vi "TestCellUtil.vi"() -> ()   [LabVIEW 2013]
doc: "This setup utility detects the NI Embedded Evaluation Kit hardware on your network and tests the configuration."
uses:
  types/TabStateType.ctl
  Controls/Refs.ctl
  Controls/Button Refs.ctl
  Controls/Tab Ctl Refs.ctl
  Controls/Indicator Refs.ctl
  Controls/Slider Refs.ctl
  Controls/Control Refs.ctl
  Controls/Network Settings.ctl
  types/UserStateType.ctl
  types/ExecutionStateType.ctl
  Controls/Detected.ctl
  Controls/Targets.ctl
  types/MAX Sys Cfg Target Information.ctl
  types/ButtonStateType.ctl
  globals/Globals.vi
  <vilib>/Platform/browser.llb/Open URL in Default Browser (string).vi
  <vilib>/regexp/Match Regular Expression.xnode
panel:
  in  "Tab Control":T1
  out "Welcome":string="Welcome to the Test Cell Controller Setup"
  out "Welcome Message":string="This wizard helps to ensure that your hardware is connected and configured properly to be used as a target in a NI VeriStand system definition.\n\n\nNote: During setup and also during the tutorials, your firewall software may prompt you to block or unblock the National Instruments software.  Select unblock whenever you encounter this prompt."
  out "Instructions":string="Connect Your Test Cell Controller Hardware"
  out "Instructions 2":string="1. Connect the Ethernet cable.\n2. Connect the power cable and press the power button.\n3. Ensure the power LED is on.\n4. Wait 20 seconds for the Test Cell Controller to boot."
  out "Detect Message":string="Click the button below to find the hardware you just connected."
  in  "Begin Detection":bool
  out "Detecting":string="Detecting Hardware\n\nSearching for Test Cell Controllers..."
  out "Detecting 2":i8(slide)=1 scale=0.0..20.0
  in  "IP Troubleshoot 2":bool
  in  "Rescan Targets":bool
  out "Detect Result Tabs":T2(tab)=enum."Found 1"
  out "Found 0 Msg":string="1. Ensure your Test Cell Controller is connected properly.\n2. Restart the Test Cell Controller by pressing the reset button (see image to left for reset button location).\n3. Wait 20 seconds for the Test Cell Controller to boot.\n4.  Click Rescan for Targets.\n\nFor troubleshooting tips, click Troubleshoot."
  out "Found 0 Status":string="Detecting Hardware\n\nNo Test Cell Controllers detected."
  out "None Detected":i8(slide)=100 scale=0.0..100.0
  out "Found 1 Msg":string="1. Check the serial number of your Test Cell Controller (see image to left for serial number location).\n2. Verify the serial number displayed here matches that of your Test Cell Controller.\n\nIf the serial number matches, click Next.\nOtherwise, ensure your hardware is connected properly, then click Rescan for Targets."
  out "Found 1 Status":string="Detecting Hardware\n\nOne Test Cell Controller detected!"
  out "Single Detected":i8(slide)=100 scale=0.0..100.0
  out "MAC Address":string
  in  "MAC Addresses":i32(listbox)=1
  out "Found 1 Msg 2":string="1. Check the serial number of your Test Cell Controller (see image to left for serial number location).\n2. Verify a serial number displayed here matches that of your Test Cell Controller.\n3. If a serial number matches, select it and click Next. \n\nOtherwise, ensure that your hardware is connected properly, then click Rescan for Targets."
  out "Found 2+ Status":string="Detecting Hardware\n\nMultiple Test Cell Controllers detected!"
  out "Multi Detected":i8(slide)=100 scale=0.0..100.0
  out "IP Troubleshoot":string="Failure to detect the Test Cell Controller may be due to one or more of the following:\n\n1. The host computer and Test Cell Controller are on different subnets.\n2. An Ethernet switch or router is off or unplugged.\n3. An Ethernet cable is loose or defective.\n4. The Test Cell Controller was unpowered or booting during the scan.\n\nPlease check for these issues, restart the Test Cell Controller by pressing the restart button (see image to left), and wait 20 seconds for the Test Cell Controller to boot.\n\nFor further troubleshooting tips, click Help.\n\nTo retry detection, click Rescan for Targets."
  out "IP Trouble Title":string="Network Troubleshooting Tips"
  out "Deploy Message":string="Software Install Required\n\nSelect Begin Install to install to the target."
  in  "Begin Deployment":bool
  out "Connecting":string="Testing Configuration\n\nDeploying to Test Cell Controller..."
  out "Deploying":i8(slide)=1 scale=0.0..20.0
  out "Symbol":u16(ring)=2
  in  "Warning":string="Warning: Do not assign the same DNS name to multiple targets on a single network"
  out "Current DNS name:":string
  in  "DNSName":string="Test-Cell-Controller"
  in  "Rename":bool
  in  "System Restore 2":bool
  out "Target MAC Address 2":string="2F14A272" caption="MAC Address"
  out "Connecting Done":string="Testing Configuration\n\nTarget software is configured correctly"
  out "Deploy Finish":i8(slide)=100 scale=0.0..100.0
  in  "Launch proj wiz":bool
  out "Complete":string="Setup Complete"
  out "Success 2":string="1. Please record the Test Cell Controller's IP Address (displayed above). It is needed for use in NI VeriStand.\n2. Click Exit Setup and Launch New Project Wizard to create a new Test Cell Controller Project."
  out "IP Address":string="10.0.42.188"
  in  "Help":bool
  out "DHCP Tabs":enum32{"IP Assignment", "DHCP", "Manual IP"}(tab)
  out "Net Setup":string="Networking Setup and Software Installation\n"
  in  "Static IP":bool
  out "DHCP Failed Tab":enum32{"Failed", "Blank"}(tab)=enum."Blank"
  out "IP Err1":string="Go back to Step 2 and check configuration."
  in  "DHCP":bool
  out "Auto IP":string="Automatic: If your Test Cell Controller is connected to your host PC through an Ethernet switch or router, select Automatic IP to request an IP address via DHCP. Contact your network administrator if your network does not support DHCP."
  in  "Default Gateway":string="10.1.128.1"
  in  "DNS Server":string="130.164.12.8"
  in  "Subnet Mask":string="255.255.254.0"
  in  "Target IP Address":string="10.1.128.143"
  out "Manual IP":string="Static (Advanced): If your Test Cell Controller is connected to your host PC directly, enter the appropriate network information below and select Static IP."
  out "Manual IP Failed Tab":enum32{"Failed", "Blank"}(tab)=enum."Blank"
  out "IP Err2":string="Go back to Step 2 and check configuration."
  out "DHCP Message":string="Configuring Test Cell Controller IP Address\n\nAttempting Automatic IP Assignment..."
  out "Assigning Auto":i8(slide)=6 scale=0.0..20.0
  out "Restore Time Note 2":string="Please be patient, this may take several minutes."
  out "Manual IP Message":string="Configuring Test Cell Controller IP Address\n\nAttempting Manual IP Assignment..."
  out "Assigning Manual":i8(slide)=6 scale=0.0..20.0
  out "Restore Time Note 3":string="Please be patient, this may take several minutes."
  out "Trouble Message 2":string="Deployment Failed"
  out "Trouble Warning":string="Restoring the target will erase all existing software on the target and may take several minutes. Please confirm that the serial number below matches the serial number printed on the target to be restored.\n\nNote: To be detected after restoration, the target must be located on the same subnet as the host computer."
  out "Trouble Message":string="1. Please reset the Test Cell Controller (see image below) and wait 20 seconds.\n2. Select Previous, then select Rescan for Targets. \n3. If deployment fails multiple times, select Restore Target System to reformat the Test Cell Controller and reimage it with the necessary software. "
  in  "System Restore":bool
  out "Target MAC Address":string="2F14A272"
  out "Reimage Tabs":enum32{"Running", "Success", "Failure"}(tab)
  out "Restore Time Note":string="Please be patient, this may take several minutes."
  out "Reimaging Tabs":enum32{"Reformat", "Reimage", "IP Config"}(tab)=enum."Reimage"
  out "Reformatting":string="Restoring Test Cell Controller\n\nReformatting ..."
  out "Reimaging":string="Installing Test Cell Controller Software\n\nCopying files ..."
  out "Auto IP Message":string="Configuring Test Cell Controller IP Address\n\nAttempting Automatic IP Assignment..."
  out "Restoring 2":i8(slide)=1 scale=0.0..20.0
  out "Restoring":i8(slide)=3 scale=0.0..20.0
  in  "Redeploy":bool
  out "Reimage Success Msg":string="The Test Cell Controller has been successfully restored."
  out "Reimage Success":string="Installing Test Cell Controller Software\n\nSuccess!"
  out "Install Success":i8(slide)=20 scale=0.0..20.0
  out "Reimage Failure":string="Installing Test Cell Controller Software\n\nFailed."
  out "Restore Failed":i8(slide)=20 scale=0.0..20.0
  out "Reimage Failure Msg":string="Your target did not reimage properly.\nPlease double-check your configuration and then contact support."
  out "Error Details:":errorcluster={"status"=TRUE, "code"=-2147220616, "source"="nisyscfg.lvlib:Get System Experts.vi:1<APPEND>\n\n<b>Complete call chain:</b>\r\n     nisyscfg.lvlib:Get System Experts.vi:1\r\n     nisyscfg.lvlib:Initialize (String).vi:1\r\n     RunDetection.vi\r\n     EvalUtil.vi"}
  out "Generic Error":string="      Unhandled Error Detected\n\nEnsure the Test Cell Controller is connected properly and reset it.  Then select Previous to retry the operation.  If the operation continues to fail, contact National Instruments for support at (866) 275-6964."
  in  "Skip Man":bool
  out "Congrats":string="Congratulations!"
  out "Success 1":string="Your Test Cell Controller has been successfully configured!\n\nIf you are new to using NI VeriStand, select Launch Getting Started Manual.  Otherwise, select Skip Manual."
  in  "GetStart Man":bool
  out "RenamingText":string="Renaming Test Cell Controller\n\nPlease be patient, this may take a minute."
  out "Renaming":i8(slide)=1 scale=0.0..20.0
  out "Main Title":string="National Instruments Test Cell Controller Setup"
  out "Step 5":string="Step 5:\nComplete"
  out "Step 4":string="Step 4:\nTarget Setup"
  out "Step 3":string="Step 3:\nHardware Detection"
  out "Step 2":string="Step 2:\nHardware Setup"
  out "Step 1":string="Step 1:\nWelcome"
  out "Skip deploy":bool
  out "LED 5":bool
  out "LED 4":bool
  out "LED 3":bool
  out "LED 2":bool
  out "LED 1":bool=TRUE
  out "Main Progress":u8(slide) scale=0.0..100.0
  in  "Exit":bool
  in  "Next":bool
  in  "Prev":bool
  in  "error in (no error)":errorcluster
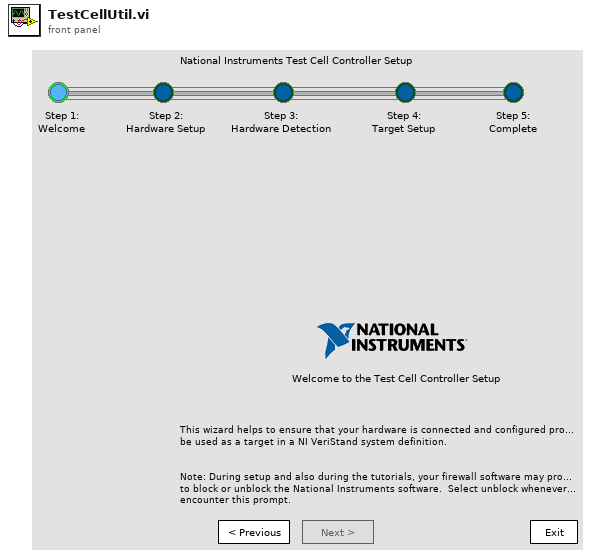
[diagram p1: front panel]
types:
  T1 = typedef "TabStateType.ctl" = enum32{"Welcome", "Instructions", "Detect", "Run Detection", "Detect Result", "Deploy", "Run Deployment", "Connect Verify", "Success", "DHCP", "Troubleshoot", "System Restore", "Error", "Video", "Rename"}
  T2 = enum32{"Found 0", "Found 1", "Found 2", "Found 3"}
  T3 = typedef "Targets.ctl" = cluster{"Dectected":T4, "Filtered Targets":T5[]}
  T4 = typedef "Detected.ctl" = enum16{"None", "Failed", "Single", "Multi"}
  T5 = typedef "MAX Sys Cfg Target Information.ctl" = cluster{"MAC Address":string, "IP Address":string, "Status":string, "Product Name":string, "Hostname":string, "Firmware/Safe Mode":string, "Subnet Mask":string, "Gateway":string, "DNS Server":string, "Serial Number":string, "Product ID":u32, "Locked ":bool, "LocalSubnet":bool, "Halt If TCP/IP Fails":bool, "Password Protected Reset":bool, "IP Mode":i32}
  T6 = typedef "ExecutionStateType.ctl" = enum16{"Init", "Welcome", "Idle", "Detect", "Run Detection", "Detect Fail", "Detect One", "Detect Mult", "Deploy", "DHCP", "Static IP", "Run Deployment", "Connect Verify", "Exit", "Video Wait", "Success", "Troubleshoot", "Troubleshoot 2", "RenameDNS"}
  T7 = typedef "UserStateType.ctl" = enum16{"Welcome", "Instructions", "Detect", "Deploy", "Success"}
  T8 = typedef "Network Settings.ctl" = cluster{"Image by default?":bool, "Working IP Config known?":bool, "DHCP?":bool}
  T9 = typedef "Refs.ctl" = cluster{"Button Refs":T10, "Tab Ctl Refs":T11, "Indicator Refs":T12, "Slider Refs":T13, "Control Refs":T14, "Deploy Message":refnum<vi>}
  T10 = typedef "Button Refs.ctl" = cluster{"Next":refnum<vi>, "Prev":refnum<vi>, "Help":refnum<vi>, "Exit":refnum<vi>, "IP Troubleshoot":refnum<vi>, "Video":refnum<vi>, "Skip Video":refnum<vi>, "Rename":refnum<vi>}
  T11 = typedef "Tab Ctl Refs.ctl" = cluster{"Tab":refnum<vi>, "Detect Result":refnum<vi>, "DHCP":refnum<vi>, "Reimage":refnum<vi>, "Reimaging":refnum<vi>, "Manual IP Failed":refnum<vi>, "DHCP Failed":refnum<vi>}
  T12 = typedef "Indicator Refs.ctl" = cluster{"Main Progress":refnum<vi>, "LED 1":refnum<vi>, "LED 2":refnum<vi>, "LED 3":refnum<vi>, "LED 4":refnum<vi>, "LED 5":refnum<vi>, "MAC Address":refnum<vi>, "Error":refnum<vi>, "Target MAC Address":refnum<vi>, "Target MAC Address 2":refnum<vi>, "IP Address":refnum<vi>, "CurrentDNSName":refnum<vi>, "Symbol":refnum<vi>, "Warning":refnum<vi>}
  T13 = typedef "Slider Refs.ctl" = cluster{"Detecting":refnum<vi>, "Single Detected":refnum<vi>, "Multi Detected":refnum<vi>, "None Detected":refnum<vi>, "Deploying":refnum<vi>, "Deploy Finish":refnum<vi>, "Assigning Manual":refnum<vi>, "Assigning Auto":refnum<vi>, "Restoring":refnum<vi>, "Restoring 2":refnum<vi>, "Restore Success":refnum<vi>, "Restore Failed":refnum<vi>, "Renaming":refnum<vi>}
  T14 = typedef "Control Refs.ctl" = cluster{"MAC Addresses":refnum<vi>, "Target IP Address":refnum<vi>, "Subnet Mask":refnum<vi>, "DNS IP":refnum<vi>, "Default Gateway":refnum<vi>, "DNSName":refnum<vi>}
  T15 = typedef "ButtonStateType.ctl" = enum16{"No change", "No Next", "No Prev", "All Disabled", "All Enabled", "Exit Only"}
  T16 = enum8{"Enabled", "Disabled", "Disabled and Grayed Out"}
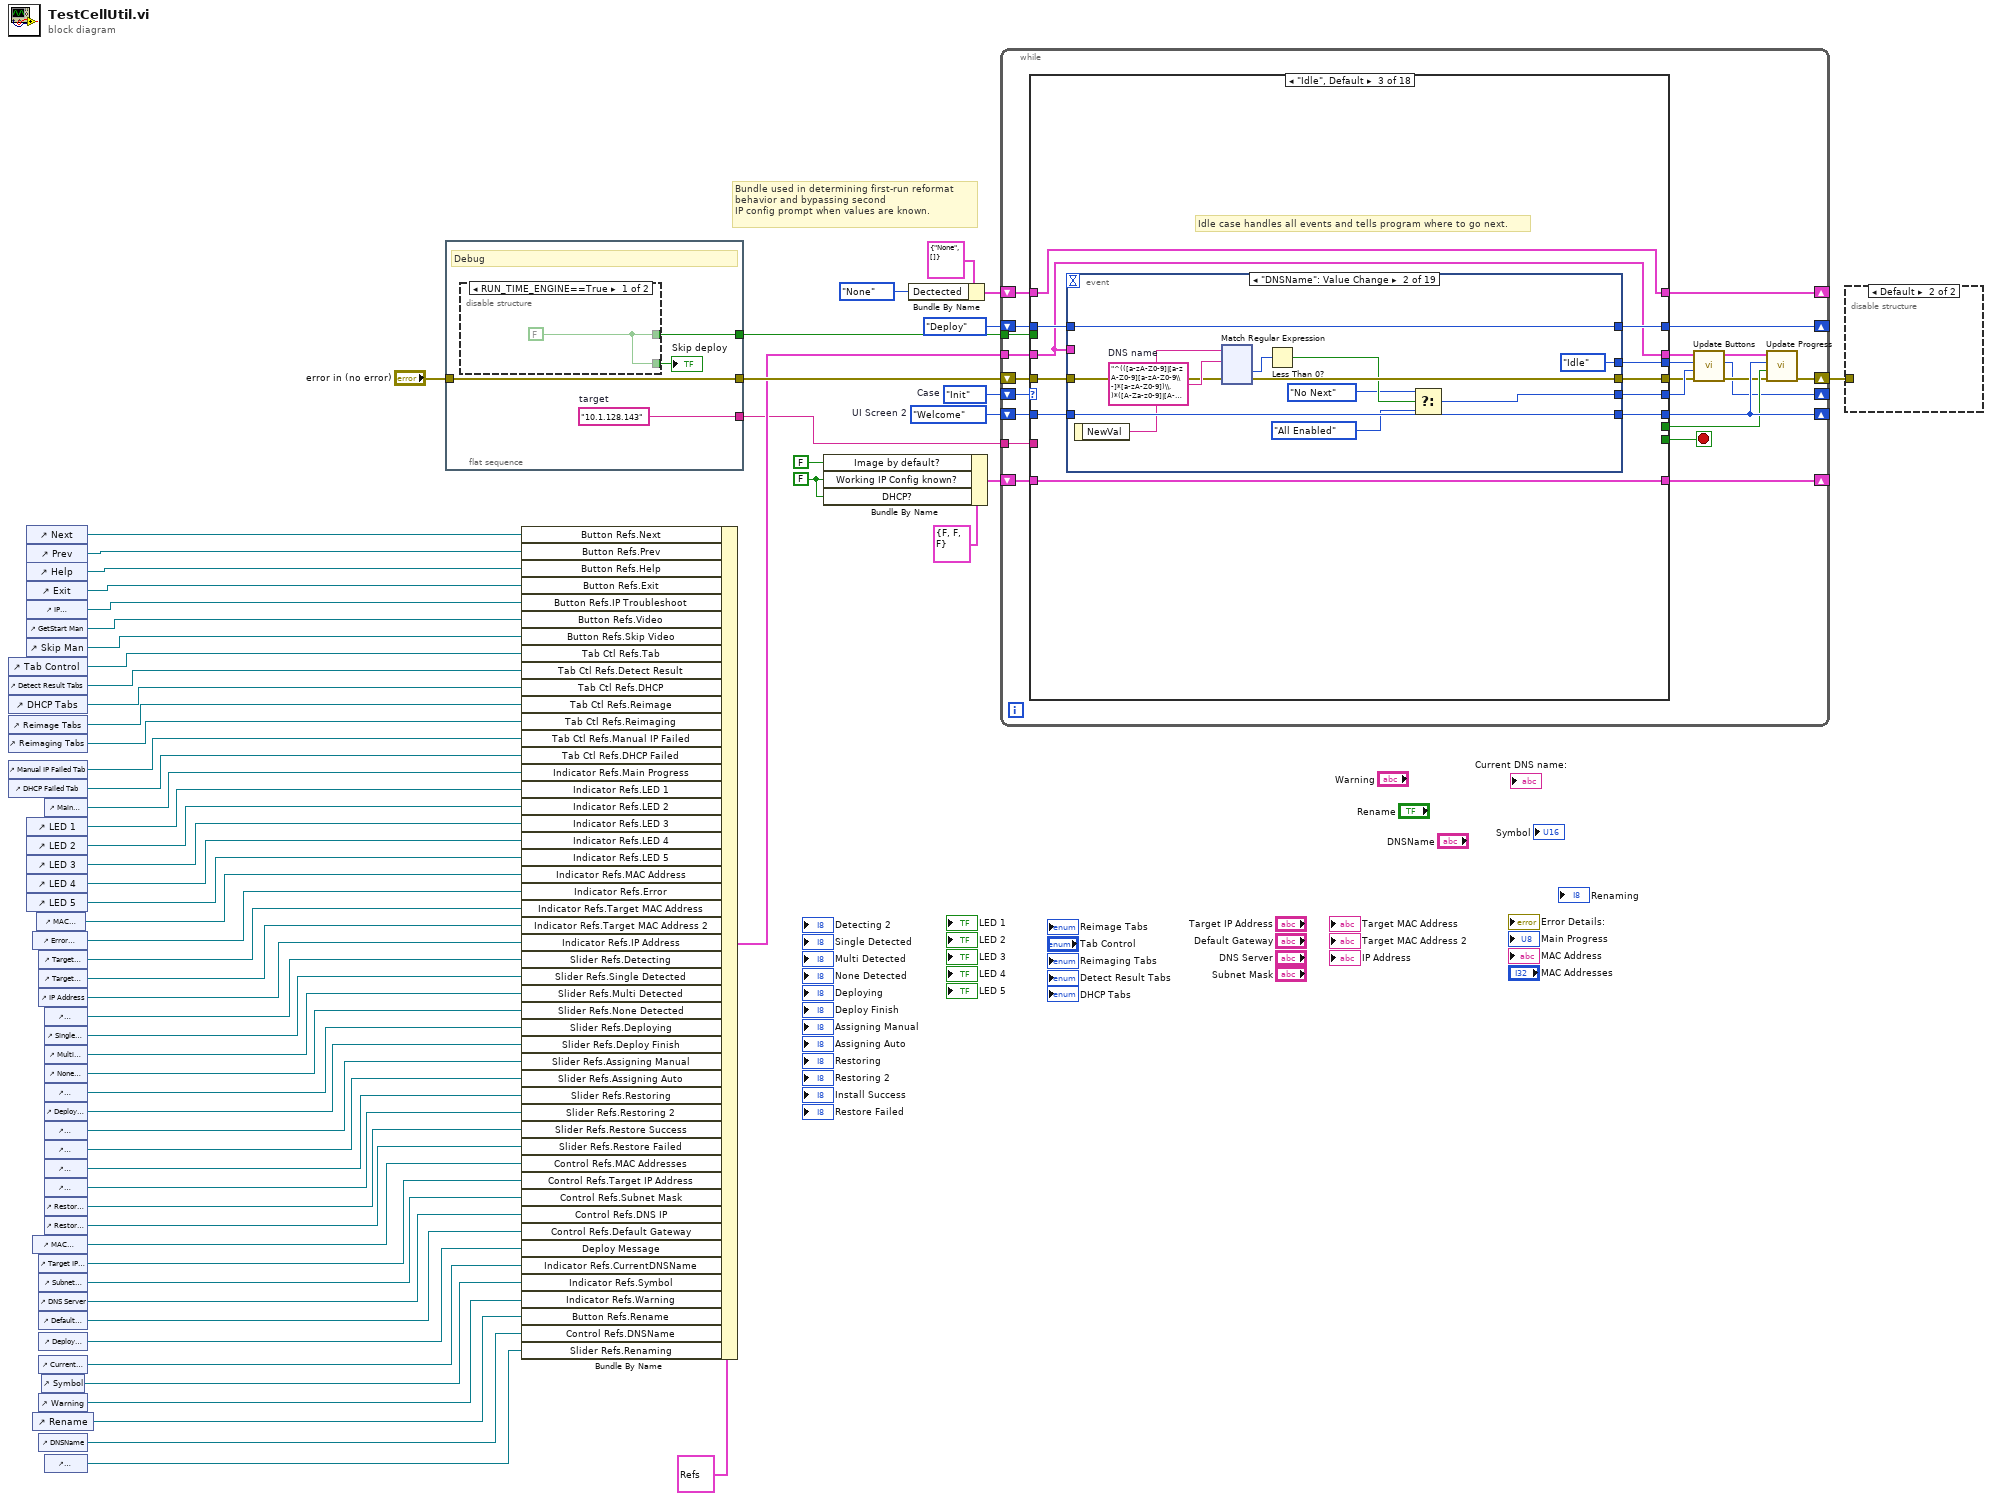
[diagram p0: block diagram]
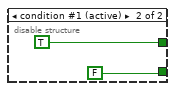
[diagram p2: hidden frame]
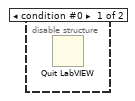
[diagram p3: hidden frame]
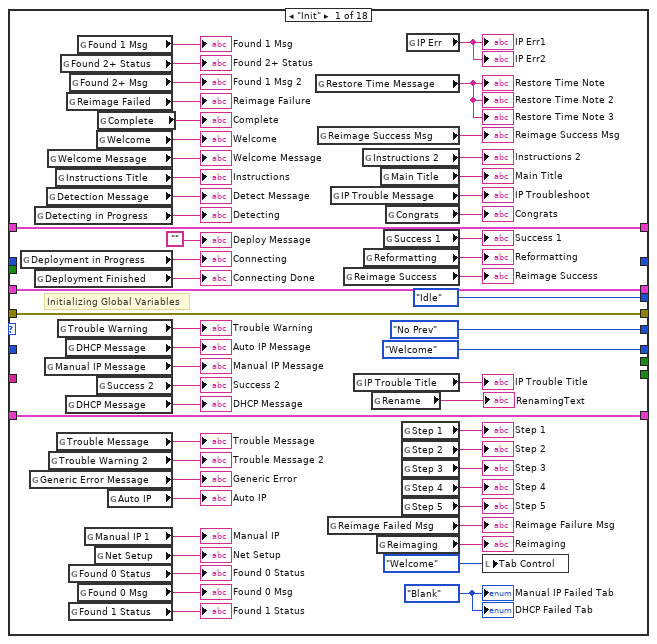
[diagram p4: hidden frame]
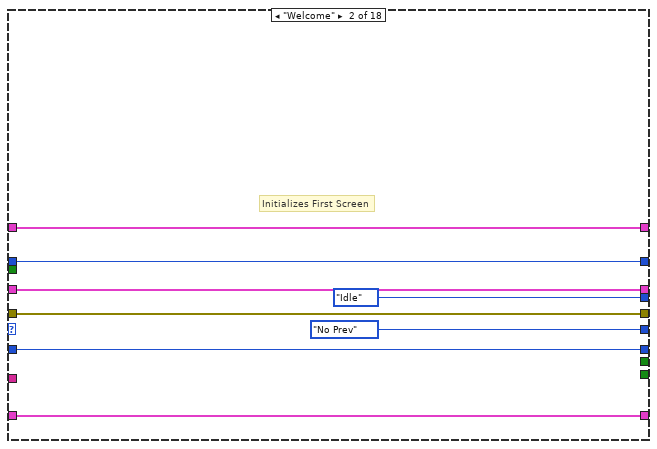
[diagram p5: hidden frame]
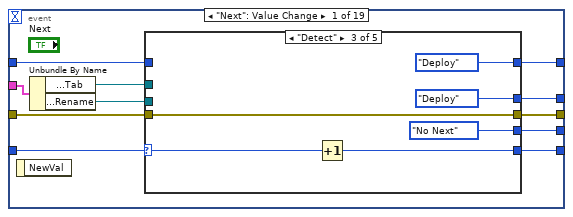
[diagram p6: hidden frame]
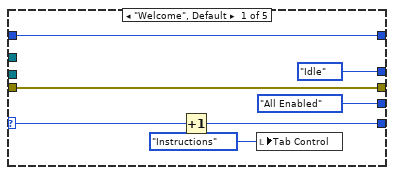
[diagram p7: hidden frame]
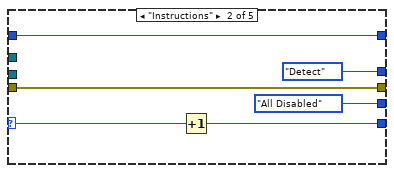
[diagram p8: hidden frame]
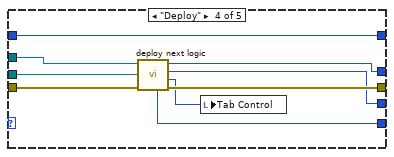
[diagram p9: hidden frame]
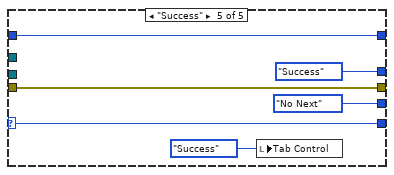
[diagram p10: hidden frame]
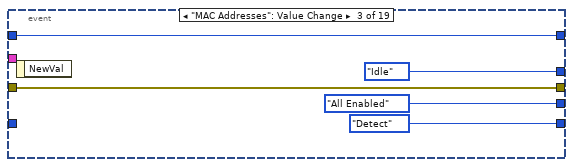
[diagram p11: hidden frame]
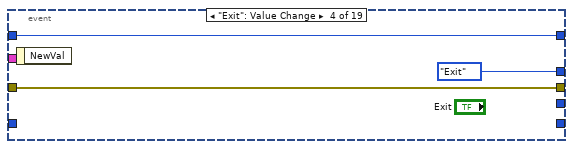
[diagram p12: hidden frame]
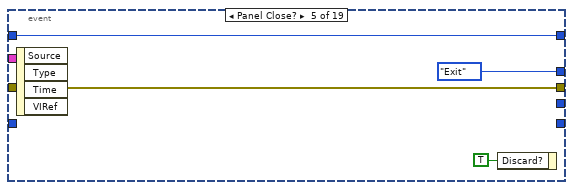
[diagram p13: hidden frame]
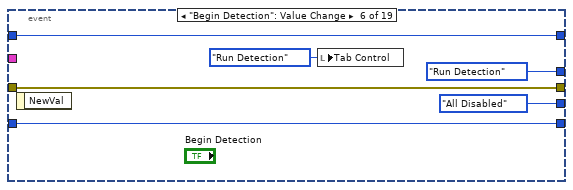
[diagram p14: hidden frame]
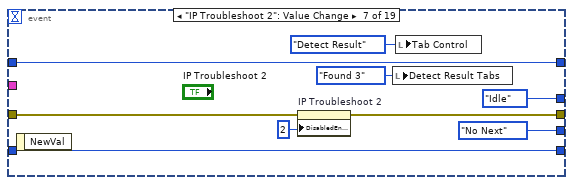
[diagram p15: hidden frame]
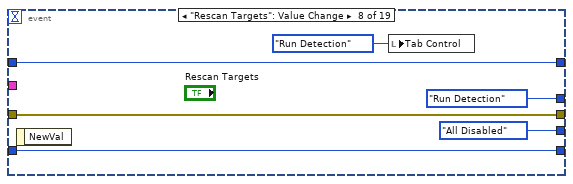
[diagram p16: hidden frame]
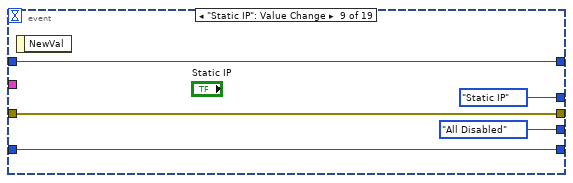
[diagram p17: hidden frame]
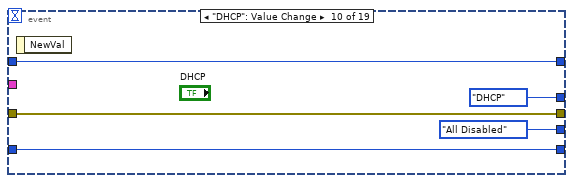
[diagram p18: hidden frame]
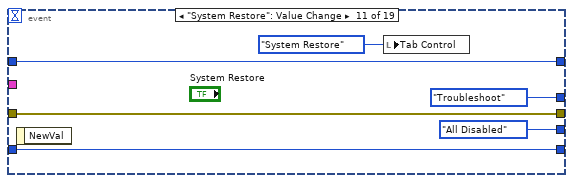
[diagram p19: hidden frame]
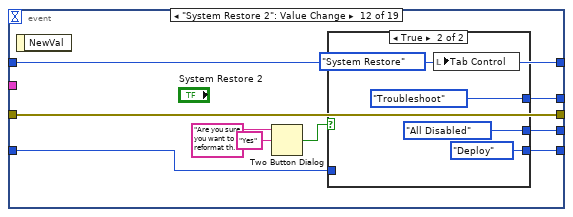
[diagram p20: hidden frame]
diagram:
  w40 = FALSE ("Working IP Config known?")
  w47 = ExecutionStateType."Init"  # Case
  w48 = UserStateType."Welcome"  # UI Screen 2
  # "Image by default?"
  # "Bundle used in determining first-run reformat\nbehavior and bypassing second\nIP config prompt when values are known."
  n1 = control-ref of="Tab Control"() -> (w58:refnum<vi>)
  n2 = control-ref of="Detect Result Tabs"() -> (w57:refnum<vi>)
  n3 = control-ref of="DHCP Tabs"() -> (w56:refnum<vi>)
  n4 = control-ref of="Reimage Tabs"() -> (w7:refnum<vi>)
  n5 = control-ref of="Reimaging Tabs"() -> (w33:refnum<vi>)
  n6 = control-ref of="Manual IP Failed Tab"() -> (w32:refnum<vi>)
  n7 = control-ref of="DHCP Failed Tab"() -> (w31:refnum<vi>)
  n8 = control-ref of="Next"() -> (w65:refnum<vi>)
  n9 = control-ref of="Prev"() -> (w64:refnum<vi>)
  n10 = control-ref of="Help"() -> (w63:refnum<vi>)
  n11 = control-ref of="Exit"() -> (w62:refnum<vi>)
  n12 = control-ref of="IP Troubleshoot 2"() -> (w61:refnum<vi>)
  n13 = control-ref of="GetStart Man"() -> (w60:refnum<vi>)
  n14 = control-ref of="Skip Man"() -> (w59:refnum<vi>)
  n15 = control-ref of="LED 1"() -> (w54:refnum<vi>)
  n16 = control-ref of="LED 2"() -> (w53:refnum<vi>)
  n17 = control-ref of="LED 3"() -> (w52:refnum<vi>)
  n18 = control-ref of="LED 4"() -> (w51:refnum<vi>)
  n19 = control-ref of="LED 5"() -> (w50:refnum<vi>)
  n20 = control-ref of="Error Details:"() -> (w38:refnum<vi>)
  n21 = control-ref of="MAC Addresses"() -> (w17:refnum<vi>)
  n22 = control-ref of="Rename"() -> (w3:refnum<vi>)
  n23 = control-ref of="MAC Address"() -> (w49:refnum<vi>)
  n24 = control-ref of="Target MAC Address"() -> (w20:refnum<vi>)
  n25 = control-ref of="Target MAC Address 2"() -> (w19:refnum<vi>)
  n26 = control-ref of="IP Address"() -> (w18:refnum<vi>)
  n27 = control-ref of="Target IP Address"() -> (w16:refnum<vi>)
  n28 = control-ref of="Subnet Mask"() -> (w15:refnum<vi>)
  n29 = control-ref of="DNS Server"() -> (w14:refnum<vi>)
  n30 = control-ref of="Default Gateway"() -> (w13:refnum<vi>)
  n31 = control-ref of="Deploy Message"() -> (w8:refnum<vi>)
  n32 = control-ref of="Current DNS name:"() -> (w6:refnum<vi>)
  n33 = control-ref of="Warning"() -> (w4:refnum<vi>)
  n34 = control-ref of="DNSName"() -> (w2:refnum<vi>)
  n35 = control-ref of="Symbol"() -> (w5:refnum<vi>)
  n36 = control-ref of="Main Progress"() -> (w55:refnum<vi>)
  n37 = control-ref of="Detecting 2"() -> (w12:refnum<vi>)
  n38 = control-ref of="Single Detected"() -> (w30:refnum<vi>)
  n39 = control-ref of="Multi Detected"() -> (w29:refnum<vi>)
  n40 = control-ref of="None Detected"() -> (w28:refnum<vi>)
  n41 = control-ref of="Deploying"() -> (w27:refnum<vi>)
  n42 = control-ref of="Deploy Finish"() -> (w26:refnum<vi>)
  n43 = control-ref of="Assigning Manual"() -> (w25:refnum<vi>)
  n44 = control-ref of="Assigning Auto"() -> (w24:refnum<vi>)
  n45 = control-ref of="Restoring"() -> (w23:refnum<vi>)
  n46 = control-ref of="Restoring 2"() -> (w9:refnum<vi>)
  n47 = control-ref of="Restore Success"() -> (w22:refnum<vi>)
  n48 = control-ref of="Restore Failed"() -> (w21:refnum<vi>)
  n49 = control-ref of="Renaming"() -> (w1:refnum<vi>)
  n50 = flat-sequence {
    tunnel: [w70] -> w44
    tunnel: "error in (no error)" -> [w70]
    tunnel: [w68] -> w11
    tunnel: [w69] -> w10
    frame #0 {
      w69 = "10.1.128.143"  # target
      # "Debug"
      n51 = disable-structure shown="RUN_TIME_ENGINE==True" {
        disable-tunnel: [w71 TRUE ("Software-Only?")] -> w68
        disable-tunnel: [w71 FALSE ("Skip deploy")] -> w67
        frame condition #0 {
          w71 = FALSE ("Software-Only?")
        }
        frame condition #1 (active) {
        }
      }
      "Skip deploy" <- w67
    }
  }
  n52 = Bundle By Name(cluster=T9 {"Button Refs"={"Next"=refnum, "Prev"=refnum, "Help"=refnum, "Exit"=refnum, "IP Troubleshoot"=refnum, "Video"=refnum, "Skip Video"=refnum, "Rename"=refnum}, "Tab Ctl Refs"={"Tab"=refnum, "Detect Result"=refnum, "DHCP"=refnum, "Reimage"=refnum, "Reimaging"=refnum, "Manual IP Failed"=refnum, "DHCP Failed"=refnum}, "Indicator Refs"={"Main Progress"=refnum, "LED 1"=refnum, "LED 2"=refnum, "LED 3"=refnum, "LED 4"=refnum, "LED 5"=refnum, "MAC Address"=refnum, "Error"=refnum, "Target MAC Address"=refnum, "Target MAC Address 2"=refnum, "IP Address"=refnum, "CurrentDNSName"=refnum, "Symbol"=refnum, "Warning"=refnum}, "Slider Refs"={"Detecting"=refnum, "Single Detected"=refnum, "Multi Detected"=refnum, "None Detected"=refnum, "Deploying"=refnum, "Deploy Finish"=refnum, "Assigning Manual"=refnum, "Assigning Auto"=refnum, "Restoring"=refnum, "Restoring 2"=refnum, "Restore Success"=refnum, "Restore Failed"=refnum, "Renaming"=refnum}, "Control Refs"={"MAC Addresses"=refnum, "Target IP Address"=refnum, "Subnet Mask"=refnum, "DNS IP"=refnum, "Default Gateway"=refnum, "DNSName"=refnum}, "Deploy Message"=refnum} ("Ctl Refs"), "Button Refs.Next"=w65, "Button Refs.Prev"=w64, "Button Refs.Help"=w63, "Button Refs.Exit"=w62, "Button Refs.IP Troubleshoot"=w61, "Button Refs.Video"=w60, "Button Refs.Skip Video"=w59, "Tab Ctl Refs.Tab"=w58, "Tab Ctl Refs.Detect Result"=w57, "Tab Ctl Refs.DHCP"=w56, "Tab Ctl Refs.Reimage"=w7, "Tab Ctl Refs.Reimaging"=w33, "Tab Ctl Refs.Manual IP Failed"=w32, "Tab Ctl Refs.DHCP Failed"=w31, "Indicator Refs.Main Progress"=w55, "Indicator Refs.LED 1"=w54, "Indicator Refs.LED 2"=w53, "Indicator Refs.LED 3"=w52, "Indicator Refs.LED 4"=w51, "Indicator Refs.LED 5"=w50, "Indicator Refs.MAC Address"=w49, "Indicator Refs.Error"=w38, "Indicator Refs.Target MAC Address"=w20, "Indicator Refs.Target MAC Address 2"=w19, "Indicator Refs.IP Address"=w18, "Slider Refs.Detecting"=w12, "Slider Refs.Single Detected"=w30, "Slider Refs.Multi Detected"=w29, "Slider Refs.None Detected"=w28, "Slider Refs.Deploying"=w27, "Slider Refs.Deploy Finish"=w26, "Slider Refs.Assigning Manual"=w25, "Slider Refs.Assigning Auto"=w24, "Slider Refs.Restoring"=w23, "Slider Refs.Restoring 2"=w9, "Slider Refs.Restore Success"=w22, "Slider Refs.Restore Failed"=w21, "Control Refs.MAC Addresses"=w17, "Control Refs.Target IP Address"=w16, "Control Refs.Subnet Mask"=w15, "Control Refs.DNS IP"=w14, "Control Refs.Default Gateway"=w13, "Deploy Message"=w8, "Indicator Refs.CurrentDNSName"=w6, "Indicator Refs.Symbol"=w5, "Indicator Refs.Warning"=w4, "Button Refs.Rename"=w3, "Control Refs.DNSName"=w2, "Slider Refs.Renaming"=w1) -> (w34:T9)
  n53 = Bundle By Name(cluster=T8 {"Image by default?"=FALSE, "Working IP Config known?"=FALSE, "DHCP?"=FALSE} ("Network Settings"), "Image by default?"=FALSE, "Working IP Config known?"=w40, "DHCP?"=w40) -> (w39:T8)
  n54 = Bundle By Name(cluster=T3 {"Dectected"=enum."None", "Filtered Targets"=[]} ("Targets"), "Dectected"=Detected."None") -> (w35:T3)
  n55 = while {
    shift-right: [w82] -> w43
    shift-left: w44 -> [w96]
    shift-right: [w89] -> _
    shift-left: w48 -> [w95]
    shift-right: [w77] -> _
    shift-left: w47 -> [w74]
    shift-right: [w81] -> _
    shift-left: w35 -> [w94]
    shift-right: [w92] -> _
    shift-left: enum16{"Deploy", "Troubleshoot"}."Deploy" -> [w93]
    shift-right: [w78] -> _
    shift-left: w39 -> [w90]
    tunnel: w34 -> [w80]
    tunnel: w11 -> [w76]
    tunnel: w10 -> [w75]
    stop <- w91 stop-if-true
    n56 = case shown="\"Idle\", Default" w74 {
      selector: w74 -> [_ _ _ _ _ _ _ _ _ w569 _ _ _ _ _ _ _ _]
      tunnel: [UserStateType."Welcome" ("Enum 2") w156 w170 UserStateType."Detect" ("Enum 2") w516 w529 w538 w549 UserStateType."Deploy" ("Enum 2") UserStateType."Deploy" ("Enum 2") UserStateType."Deploy" ("Enum 2") w593 w600 w609 w620 UserStateType."Deploy" ("Enum 2") w641 w646] -> w89
      tunnel: w96 -> [w99 w159 w169 w502 w517 w527 w537 w548 w559 w574 w584 w588 w595 w604 w617 w634 w644 w655]
      tunnel: [w99 w159 w168 w504 w515 w526 w534 w543 w562 w572 w585 w587 w595 w605 w616 w631 w643 w654] -> w83
      tunnel: [_ _ _ _ _ _ _ _ _ _ _ _ TRUE _ _ _ _ _] -> w91
      tunnel: [ButtonStateType."No Prev" ("Enum") ButtonStateType."No Prev" ("Enum") w167 ButtonStateType."All Disabled" ("Enum") ButtonStateType."All Disabled" ("Enum") w525 ButtonStateType."All Enabled" ("Enum") ButtonStateType."No Next" ("Enum") w560 w573 w582 w591 ButtonStateType."No Next" ("Enum") ButtonStateType."No Next" ("Enum") ButtonStateType."No change" ("Enum") w630 ButtonStateType."No Next" ("Enum") w648] -> w85
      tunnel: w95 -> [_ w156 w166 _ w516 w529 w538 w549 _ _ _ w593 w600 w609 w620 _ _ w650]
      tunnel: [ExecutionStateType."Idle" ("Enum") ExecutionStateType."Idle" ("Enum") w165 w501 w513 ExecutionStateType."Idle" ("Enum") ExecutionStateType."Idle" ("Enum") ExecutionStateType."Idle" ("Enum") w552 w570 w577 w592 ExecutionStateType."Idle" ("Enum") ExecutionStateType."Idle" ("Enum") ExecutionStateType."Idle" ("Enum") w629 w639 w649] -> w84
      tunnel: w94 -> [w148 w155 w162 w499 w511 w521 w532 w541 w556 w567 w580 w586 w597 w611 w614 w626 w636 w652]
      tunnel: [w148 w155 w162 w497 w509 w519 w530 w544 w555 w564 w578 w586 w597 w611 w612 w623 w635 w651] -> w81
      tunnel: [_ _ _ _ _ _ _ _ _ _ _ _ _ _ _ TRUE TRUE _] -> w88
      tunnel: [_ w154 w164 _ _ _ _ _ w561 w571 _ _ _ w607 _ w628 _ w647] -> w92
      tunnel: w93 -> [_ w154 w163 _ _ _ _ _ w561 w571 _ _ _ w607 _ _ _ w647]
      tunnel: w90 -> [w107 w153 w161 w503 w514 w524 w535 w545 w553 w566 w583 w590 w596 w606 w618 w625 w640 w656]
      tunnel: [w107 w153 w161 w503 w514 w524 w535 w545 w554 w563 w583 w590 w596 w606 w618 w622 w640 w656] -> w78
      tunnel: w80 -> [w101 w152 w160 w500 w512 w522 w533 w542 w558 w568 w581 w589 w594 w603 w615 w627 w638 w653]
      tunnel: [w101 w152 w160 w498 w510 w520 w531 w540 w557 w565 w579 w589 w594 w602 w613 w624 w637 w653] -> w79
      tunnel: w76 -> [_ _ _ _ w507 _ _ _ _ _ _ _ _ _ _ _ _ _]
      tunnel: w75 -> [_ _ _ _ w508 _ _ _ _ _ _ _ _ _ _ _ _ _]
      frame "Init" {
        w126 = enum32{"Failed", "Blank"}."Blank" ("DHCP Failed Tab")
        # "Initializing Global Variables"
        n57 = global read "Globals.vi" "Deployment in Progress"() -> (→"Connecting":string)
        n58 = global read "Globals.vi" "Generic Error Message"() -> (→"Generic Error":string)
        n59 = global read "Globals.vi" "Detecting in Progress"() -> (→"Detecting":string)
        n60 = global read "Globals.vi" "Deployment Finished"() -> (→"Connecting Done":string)
        n61 = global read "Globals.vi" "Manual IP Message"() -> (→"Manual IP Message":string)
        n62 = global read "Globals.vi" "Detection Message"() -> (→"Detect Message":string)
        n63 = global read "Globals.vi" "Welcome Message"() -> (→"Welcome Message":string)
        n64 = global read "Globals.vi" "Trouble Warning 2"() -> (→"Trouble Message 2":string)
        n65 = global read "Globals.vi" "Instructions Title"() -> (→"Instructions":string)
        n66 = global read "Globals.vi" "Trouble Message"() -> (→"Trouble Message":string)
        n67 = global read "Globals.vi" "Trouble Warning"() -> (→"Trouble Warning":string)
        n68 = global read "Globals.vi" "Found 2+ Status"() -> (→"Found 2+ Status":string)
        n69 = global read "Globals.vi" "DHCP Message"() -> (→"Auto IP Message":string)
        n70 = global read "Globals.vi" "DHCP Message"() -> (→"DHCP Message":string)
        n71 = global read "Globals.vi" "Reimage Failed"() -> (→"Reimage Failure":string)
        n72 = global read "Globals.vi" "Found 0 Status"() -> (→"Found 0 Status":string)
        n73 = global read "Globals.vi" "Found 1 Status"() -> (→"Found 1 Status":string)
        n74 = global read "Globals.vi" "Found 2+ Msg"() -> (→"Found 1 Msg 2":string)
        n75 = global read "Globals.vi" "Found 1 Msg"() -> (→"Found 1 Msg":string)
        n76 = global read "Globals.vi" "Found 0 Msg"() -> (→"Found 0 Msg":string)
        n77 = global read "Globals.vi" "Manual IP 1"() -> (→"Manual IP":string)
        n78 = global read "Globals.vi" "Net Setup"() -> (→"Net Setup":string)
        n79 = global read "Globals.vi" "Welcome"() -> (→"Welcome":string)
        n80 = global read "Globals.vi" "Success 2"() -> (→"Success 2":string)
        n81 = global read "Globals.vi" "Complete"() -> (→"Complete":string)
        n82 = global read "Globals.vi" "Auto IP"() -> (→"Auto IP":string)
        n83 = global read "Globals.vi" "Restore Time Message"() -> (→"Restore Time Note" →"Restore Time Note 3" →"Restore Time Note 2":string)
        n84 = global read "Globals.vi" "Reimage Success Msg"() -> (→"Reimage Success Msg":string)
        n85 = global read "Globals.vi" "Reimage Failed Msg"() -> (→"Reimage Failure Msg":string)
        n86 = global read "Globals.vi" "IP Trouble Message"() -> (→"IP Troubleshoot":string)
        n87 = global read "Globals.vi" "Reimage Success"() -> (→"Reimage Success":string)
        n88 = global read "Globals.vi" "IP Trouble Title"() -> (→"IP Trouble Title":string)
        n89 = global read "Globals.vi" "Instructions 2"() -> (→"Instructions 2":string)
        n90 = global read "Globals.vi" "Reformatting"() -> (→"Reformatting":string)
        n91 = global read "Globals.vi" "Rename"() -> (→"RenamingText":string)
        n92 = global read "Globals.vi" "Reimaging"() -> (→"Reimaging":string)
        n93 = global read "Globals.vi" "Main Title"() -> (→"Main Title":string)
        n94 = global read "Globals.vi" "Success 1"() -> (→"Success 1":string)
        n95 = global read "Globals.vi" "Congrats"() -> (→"Congrats":string)
        n96 = global read "Globals.vi" "Step 1"() -> (→"Step 1":string)
        n97 = global read "Globals.vi" "Step 2"() -> (→"Step 2":string)
        n98 = global read "Globals.vi" "Step 3"() -> (→"Step 3":string)
        n99 = global read "Globals.vi" "Step 4"() -> (→"Step 4":string)
        n100 = global read "Globals.vi" "Step 5"() -> (→"Step 5":string)
        n101 = global read "Globals.vi" "IP Err"() -> (→"IP Err2" →"IP Err1":string)
        n102 = local write "Tab Control"(TabStateType."Welcome" ("Tab Control")) -> ()
        "Deploy Message" <- ""
        "DHCP Failed Tab" <- w126
        "Manual IP Failed Tab" <- w126
      }
      frame "Welcome" {
        # "Initializes First Screen"
      }
      frame "Idle", Default {
        # "Idle case handles all events and tells program where to go next."
        n103 = event shown="[1] \"DNSName\": Value Change" {
          selector: _ -> [_ _ _ _ _ _ _ _ _ _ _ _ _ _ _ _ _ _ _]
          dyn-events: _ -> [_ _ _ _ _ _ _ _ _ _ _ _ _ _ _ _ _ _ _]
          timeout: _ -> [_ _ _ _ _ _ _ _ _ _ _ _ _ _ _ _ _ _ _]
          tunnel: w166 -> [w181 w221 _ _ _ w359 w368 w374 w379 w384 w390 w391 _ w421 w427 w451 w455 w463 w488]
          tunnel: [w171 w221 UserStateType."Detect" _ _ w359 w368 w374 w379 w384 w390 w392 UserStateType."Deploy" w421 w427 w451 w455 w458 w488] -> w170
          tunnel: w169 -> [w175 w225 w344 w347 w351 w354 w361 w369 w376 w381 w385 w397 w407 w416 w425 w452 w454 w459 w495]
          tunnel: [w173 w224 w344 w347 w351 w354 w360 w369 w376 w381 w385 w397 w407 w417 w422 w444 w454 w459 w492] -> w168
          tunnel: [w180 w216 ButtonStateType."All Enabled" ("Enum") _ _ ButtonStateType."All Disabled" ("Enum") ButtonStateType."No Next" ("Enum") ButtonStateType."All Disabled" ("Enum") ButtonStateType."All Disabled" ("Enum") ButtonStateType."All Disabled" ("Enum") ButtonStateType."All Disabled" ("Enum") w393 ButtonStateType."All Disabled" ("Enum") ButtonStateType."No change" ("Enum") ButtonStateType."All Disabled" ("Enum") ButtonStateType."No change" ("Enum") ButtonStateType."No Next" ("Enum") w462 ButtonStateType."No change" ("Enum")] -> w167
          tunnel: [w179 ExecutionStateType."Idle" ("Enum") ExecutionStateType."Idle" ("Enum") ExecutionStateType."Exit" ("Enum") ExecutionStateType."Exit" ("Enum") ExecutionStateType."Run Detection" ("Enum") ExecutionStateType."Idle" ("Enum") ExecutionStateType."Run Detection" ("Enum") ExecutionStateType."Static IP" ("Enum") ExecutionStateType."DHCP" ("Enum") ExecutionStateType."Troubleshoot" ("Enum") w399 ExecutionStateType."Run Deployment" ("Enum") ExecutionStateType."Idle" ("Enum") ExecutionStateType."Video Wait" ("Enum") ExecutionStateType."Idle" ("Enum") ExecutionStateType."Idle" ("Enum") w461 ExecutionStateType."Idle" ("Enum")] -> w165
          tunnel: [w178 w223 w342 w348 w352 w356 w365 w371 w375 w380 w387 w398 w410 w420 w426 w450 _ enum16{"Deploy", "Troubleshoot"}."Deploy" w491] -> w164
          tunnel: w163 -> [w177 w223 w342 w348 w352 w356 w365 w371 w375 w380 w387 w398 w410 w420 w426 w450 _ _ w491]
          tunnel: w160 -> [w176 _ _ _ _ _ _ _ _ _ _ _ _ _ _ _ _ _ w494]
          event "Next": Value Change {
            n104 = event-data() -> ()  [unwired: 2 out]
            n105 = Unbundle By Name(w176) -> ("Tab Ctl Refs.Tab"=w174:refnum<vi>, "Button Refs.Rename"=w172:refnum<vi>)
            n106 = case shown="\"Detect\"" w181 {
              selector: w181 -> [w186 w192 w198 _ w213]
              tunnel: [w182 w189 w195 w201 w213] -> w171
              tunnel: [ExecutionStateType."Idle" ("Enum") ExecutionStateType."Detect" ("Enum") ExecutionStateType."Deploy" ("Enum") w205 ExecutionStateType."Success" ("Enum")] -> w179
              tunnel: [ButtonStateType."All Enabled" ("Enum") ButtonStateType."All Disabled" ("Enum") ButtonStateType."No Next" ("Enum") w204 ButtonStateType."No Next" ("Enum")] -> w180
              tunnel: [w185 w191 enum16{"Deploy", "Troubleshoot"}."Deploy" w209 w212] -> w178
              tunnel: w177 -> [w185 w191 _ w209 w212]
              tunnel: w175 -> [w183 w190 w196 w208 w210]
              tunnel: w174 -> [_ _ _ w207 _]
              tunnel: [w183 w190 w196 w206 w210] -> w173
              tunnel: w172 -> [_ _ _ w202 _]
              frame "Welcome", Default {
                n107 = Increment(x=w186) -> (x+1=w182:T7)
                n108 = local write "Tab Control"(TabStateType."Instructions" ("Tab Control")) -> ()
              }
              frame "Instructions" {
                n109 = Increment(x=w192) -> (x+1=w189:T7)
              }
              frame "Detect" {
                n110 = Increment(x=w198) -> (x+1=w195:T7)
              }
              frame "Deploy" {
                n111 = call "deploy next logic.vi"("error in (no error)"=w208, "Rename"=w202, "TabControl in"=w207) -> ("error out"=w206:errorcluster, "Tab Control"=w203:T1, "Button state"=w204:T15, "Execution state"=w205:T6, "UI Screen out"=w201:T7)  [unwired: 4 in]
                n112 = local write "Tab Control"(w203) -> ()
              }
              frame "Success" {
                n113 = local write "Tab Control"(TabStateType."Success" ("Tab Control")) -> ()
              }
            }
          }
          event "DNSName": Value Change {
            w226 = "^(([a-zA-Z0-9]|[a-zA-Z0-9][a-zA-Z0-9\\-]*[a-zA-Z0-9])\\.)*([A-Za-z0-9]|[A-Za-z0-9][A-Za-z0-9\\-]*[A-Za-z0-9])$"  # DNS name
            n114 = event-data() -> ("NewVal"=w219:string)  [unwired: 1 out]
            n115 = xnode "Match Regular Expression"("input string"=w219, "regular expression"=w226, "error in"=w225) -> ("offset past match"=w227:i32, "error out"=w224:errorcluster)  [unwired: 3 in, 3 out]
            n116 = Less Than 0?(x=w227) -> (x < 0?=w220:bool)
            n117 = Select(t=ButtonStateType."No Next" ("Enum"), s=w220, f=ButtonStateType."All Enabled" ("Enum")) -> (s? t:f=w216:T15)
          }
          event "MAC Addresses": Value Change {
            n118 = event-data() -> ()  [unwired: 2 out]
          }
          event "Exit": Value Change {
            n119 = event-data() -> ()  [unwired: 2 out]
          }
          event Panel Close? {
            n120 = event-data() -> ()  [unwired: 5 out]
            n121 = event-data("Discard?"=TRUE) -> ()  [unwired: 1 in, 1 out]
          }
          event "Begin Detection": Value Change {
            n122 = event-data() -> ()  [unwired: 2 out]
            n123 = local write "Tab Control"(TabStateType."Run Detection" ("Tab Control")) -> ()
          }
          event "IP Troubleshoot 2": Value Change {
            n124 = event-data() -> ()  [unwired: 2 out]
            n125 = property on="IP Troubleshoot 2" class="Bool"(error in=w361, "DisabledEnum"=u8 2 ("Disabled")) -> (error out=w360:errorcluster)  [unwired: 1 in, 1 out]
            n126 = local write "Detect Result Tabs"(T2."Found 3" ("Detect Result Tabs")) -> ()
            n127 = local write "Tab Control"(TabStateType."Detect Result" ("Tab Control")) -> ()
          }
          event "Rescan Targets": Value Change {
            n128 = event-data() -> ()  [unwired: 2 out]
            n129 = local write "Tab Control"(TabStateType."Run Detection" ("Tab Control")) -> ()
          }
          event "Static IP": Value Change {
            n130 = event-data() -> ()  [unwired: 2 out]
          }
          event "DHCP": Value Change {
            n131 = event-data() -> ()  [unwired: 2 out]
          }
          event "System Restore": Value Change {
            n132 = event-data() -> ()  [unwired: 2 out]
            n133 = local write "Tab Control"(TabStateType."System Restore" ("Tab Control")) -> ()
          }
          event "System Restore 2": Value Change {
            n134 = event-data() -> ()  [unwired: 2 out]
            n135 = Two Button Dialog(message="Are you sure you want to reformat the target? This will erase all files on the target and perform a clean install. Ensure there are no important data logs or other files of value on the target.", 2:"Yes" ("T button name (\"OK\")")) -> (T button?=w394:bool)  [unwired: 1 in]
            n136 = case shown="True" w394 {
              tunnel: [ExecutionStateType."Idle" ("Enum") ExecutionStateType."Troubleshoot" ("Enum")] -> w399
              tunnel: [ButtonStateType."No change" ("Enum") ButtonStateType."All Disabled" ("Enum")] -> w393
              tunnel: [w400 UserStateType."Deploy" ("UI Screen 2")] -> w392
              tunnel: w391 -> [w400 _]
              frame False {
              }
              frame True {
                n137 = local write "Tab Control"(TabStateType."System Restore" ("Tab Control")) -> ()
              }
            }
          }
          event "Begin Deployment", "Redeploy": Value Change {
            n138 = event-data() -> ()  [unwired: 2 out]
            n139 = local write "Tab Control"(TabStateType."Run Deployment" ("Tab Control")) -> ()
          }
          event "Launch proj wiz": Value Change {
            n140 = event-data() -> ()  [unwired: 2 out]
            n141 = global read "Globals.vi" "Relative Wiz Path"() -> (w419:string)
            n142 = call "Get Document Dir.vi"() -> ("document dir"=w418:path)
            n143 = Build Path(base path=w418, name or relative path=w419) -> (appended path=w415:path)
            n144 = call "Display External Document.vi"("error in (no error)"=w416, "Document Path"=w415) -> ("error out"=w417:errorcluster)  [unwired: 9 in]
          }
          event "GetStart Man": Value Change {
            n145 = event-data() -> ()  [unwired: 2 out]
            n146 = disable-structure shown="Disabled" {
              disable-tunnel: w425 -> [w434 w442]
              disable-tunnel: [w429 w441] -> w422
              frame Disabled {
                n147 = global read "Globals.vi" "Tutorial Root Path"() -> (w433)
                n148 = Current VI's Path() -> (path=w440:path)
                n149 = global read "Globals.vi" "Video Path"() -> (w432:string)
                n150 = Build Path(base path=w440, name or relative path=w433) -> (appended path=w439:path)
                n151 = Path To String(path=w439) -> (string=w437:string)
                n152 = Concatenate Strings("cmd /C" ("command line"), "\"" ("string"), w437) -> (w435:string)
                n153 = Concatenate Strings(w435, w432) -> (w428:string)
                n154 = call <vilib>:"System Exec.vi"("run minimized? (F)"=TRUE, "wait until completion? (T)"=FALSE, "error in (no error)"=w434, "command line"=w428) -> ("error out"=w429:errorcluster)  [unwired: 2 in, 5 out]
              }
              frame Enabled {
                n155 = call-poly <vilib>:"Open URL in Default Browser.vi"("error in (no error)"=w442, "URL"="http://www.youtube.com/watch?v=Cr8SGI0AC7s&feature=player_embedded#t=0s") -> ("error out"=w441:errorcluster)  [unwired: 4 in, 1 out]
              }
            }
          }
          event "Help": Value Change {
            n156 = event-data() -> ()  [unwired: 2 out]
            n157 = global read "Globals.vi" "Relative Help Path"() -> (w447:string)
            n158 = call "Get Document Dir.vi"() -> ("document dir"=w446:path)
            n159 = Build Path(base path=w446, name or relative path=w447) -> (appended path=w445:path)
            n160 = call "Display External Document.vi"("error in (no error)"=w452, "Document Path"=w445) -> ("error out"=w444:errorcluster)  [unwired: 9 in]
          }
          event "Skip Man": Value Change {
            n161 = event-data() -> ()  [unwired: 2 out]
            n162 = local write "Tab Control"(TabStateType."Success" ("Tab Control")) -> ()
          }
          event "Prev": Value Change {
            n163 = event-data() -> ()  [unwired: 2 out]
            n164 = case shown="\"Success\"" w463 {
              selector: w463 -> [w464 w468 w473 w476 w481]
              tunnel: [w464 w466 w471 w477 w480] -> w458
              tunnel: [ExecutionStateType."Init" ("Enum") ExecutionStateType."Idle" ("Enum") ExecutionStateType."Idle" ("Enum") ExecutionStateType."Detect" ("Enum") ExecutionStateType."Detect" ("Enum")] -> w461
              tunnel: [_ ButtonStateType."No Prev" ("Enum") ButtonStateType."All Enabled" ("Enum") _ ButtonStateType."All Disabled" ("Enum")] -> w462
              frame "Welcome" {
                # "shouldnt happen"
              }
              frame "Instructions" {
                n165 = Decrement(x=w468) -> (x-1=w466:T7)
                n166 = local write "Tab Control"(TabStateType."Welcome" ("Tab Control")) -> ()
              }
              frame "Detect" {
                n167 = Decrement(x=w473) -> (x-1=w471:T7)
                n168 = local write "Tab Control"(TabStateType."Instructions" ("Tab Control")) -> ()
              }
              frame "Deploy" {
                n169 = Decrement(x=w476) -> (x-1=w477:T7)
              }
              frame "Success" {
                n170 = Decrement(x=w481) -> (x-1=w479:T7)
                n171 = Decrement(x=w479) -> (x-1=w480:T7)
              }
            }
          }
          event "Rename": Value Change {
            n172 = event-data() -> ("NewVal"=w487:bool)  [unwired: 1 out]
            n173 = Unbundle By Name(w494) -> ("Control Refs.DNSName"=w493:refnum<vi>)
            n174 = Select(t=T16."Enabled" ("Disabled"), s=w487, f=T16."Disabled and Grayed Out" ("Disabled")) -> (s? t:f=w484:T16)
            n175 = property class="Str"(reference=w493, error in=w495, "DisabledEnum"=w484) -> (error out=w492:errorcluster)  [unwired: 1 out]
          }
        }
      }
      frame "Detect" {
        # "Detecting Targets on Network"
        n176 = control-ref of="This VI"() -> (w496:refnum<vi>)
        n177 = call "Detect.vi"("VI to busy"=w496, "error in (no error)"=w502, "Targets in"=w499, "Ctl Refs in"=w500) -> ("error out"=w504:errorcluster, "Execution State"=w501:T6, "Targets out"=w497:T3, "Ctl Refs out"=w498:T9)  [unwired: 4 in]
      }
      frame "Run Detection" {
        n178 = call "Run Detection.vi"("Specific target IP"=w508, "Specific target (F)"=w507, "Reduce Discovery Timeout (T)"=w507, "error in (no error)"=w517, "Targets in"=w511, "Ctl Refs in"=w512) -> ("error out"=w515:errorcluster, "State"=w513:T6, "Targets out"=w509:T3, "Ctl Refs out"=w510:T9)  [unwired: 2 in]
      }
      frame "Detect Fail" {
        n179 = local read "Skip deploy"() -> (w523:bool)
        n180 = call "Detect Failed.vi"("error in (no error)"=w527, "Software-Only?"=w523, "Targets in"=w521, "Ctl Refs in"=w522) -> ("error out"=w526:errorcluster, "Enum"=w525:T15, "Targets out"=w519:T3, "Ctl Refs out"=w520:T9)  [unwired: 4 in]
      }
      frame "Detect One" {
        n181 = call "One Detected.vi"("error in (no error)"=w537, "Targets in"=w532, "Ctl Refs in"=w533) -> ("error out"=w534:errorcluster, "Targets out"=w530:T3, "Ctl Refs out"=w531:T9)  [unwired: 6 in]
      }
      frame "Detect Mult" {
        n182 = call "Multi Detected.vi"("error in (no error)"=w548, "Targets in"=w541, "Ctl Refs in"=w542) -> ("error out"=w543:errorcluster, "Targets out"=w544:T3, "Ctl Refs out"=w540:T9)  [unwired: 6 in]
      }
      frame "Deploy" {
        n183 = control-ref of="This VI"() -> (w550:refnum<vi>)
        n184 = call "Deploy.vi"("VI reference (current VI)"=w550, "error in (no error)"=w559, "Network Settings in"=w553, "Targets in"=w556, "Ctl Refs in"=w558) -> ("error out"=w562:errorcluster, "Network Settings out"=w554:T8, "Targets out"=w555:T3, "Ctl Refs out"=w557:T9, "Button State"=w560:T15, "Execution State"=w552:T6)  [unwired: 1 in]
      }
      frame "DHCP", "Static IP" {
        n185 = call "Change Network Settings.vi"("Execution State in"=w569, "Deploy in"=w571, "error in (no error)"=w574, "Network Settings in"=w566, "Targets in"=w567, "Ctl Refs in"=w568) -> ("error out"=w572:errorcluster, "Network Settings out"=w563:T8, "Targets out"=w564:T3, "Ctl Refs out"=w565:T9, "Buttons out"=w573:T15, "Execution State out"=w570:T6)
      }
      frame "Run Deployment" {
        n186 = call "Run Deployment.vi"("error in (no error)"=w584, "Targets in"=w580, "Ctl Refs in"=w581) -> ("error out"=w585:errorcluster, "Execution State out"=w577:T6, "Targets out"=w578:T3, "Ctl Refs out"=w579:T9, "Buttons out"=w582:T15)  [unwired: 4 in]
      }
      frame "Connect Verify" {
        n187 = call "Connect Verify.vi"("error in (no error)"=w588, "Targets in"=w586, "Ctl Refs"=w589) -> ("error out"=w587:errorcluster, "Button state"=w591:T15, "Execution state"=w592:T6)  [unwired: 6 in]
      }
      frame "Exit" {
        # "Aborts FPGA bitfile is exit button is selected"
      }
      frame "Video Wait" {
        n188 = call "Video Wait.vi"("error in (no error)"=w604, "Ctl Refs in"=w603) -> ("error out"=w605:errorcluster, "Ctl Refs out"=w602:T9)  [unwired: 8 in]
      }
      frame "Success" {
        n189 = call "Success.vi"("error in (no error)"=w617, "Targets in"=w614, "Ctl Refs in"=w615) -> ("error out"=w616:errorcluster, "Targets out"=w612:T3, "Ctl Refs out"=w613:T9)  [unwired: 6 in]
      }
      frame "Troubleshoot" {
        # "Reformats"
        n190 = call "Troubleshoot 1.vi"("error in (no error)"=w634, "Network Settings in"=w625, "Targets in"=w626, "Ctl Refs in"=w627) -> ("error out"=w631:errorcluster, "Network Settings out"=w622:T8, "Targets out"=w623:T3, "Ctl Refs out"=w624:T9, "Buttons out"=w630:T15, "Execution State"=w629:T6, "Deploy out"=w628:enum16{"Deploy", "Troubleshoot"})  [unwired: 1 in]
      }
      frame "Troubleshoot 2" {
        # "Installs software"
        n191 = call "Troubleshoot 2.vi"("error in (no error)"=w644, "Targets in"=w636, "Ctl Refs in"=w638) -> ("error out"=w643:errorcluster, "User State"=w641:T7, "Targets out"=w635:T3, "Ctl Refs out"=w637:T9, "Execution State"=w639:T6)  [unwired: 4 in]
      }
      frame "RenameDNS" {
        n192 = Increment(x=w650) -> (x+1=w646:T7)
        n193 = call "RenameDNS.vi"("error in (no error)"=w655, "Targets in"=w652, "Ctl Refs in"=w653) -> ("error out"=w654:errorcluster, "Targets out"=w651:T3, "Buttons out"=w648:T15, "Execution State out"=w649:T6)  [unwired: 5 in]
      }
    }
    n194 = call "Update Buttons.vi"("error in (no error)"=w83, "Button State"=w85, "Execution State in"=w84, "Ctl Refs in"=w79) -> ("error out"=w86:errorcluster, "Execution State out"=w77:T6, "Ctl Refs out"=w87:T9)  [unwired: 5 in]
    n195 = call "Update Progress.vi"("error in (no error)"=w86, "Troubleshoot?"=w88, "User State"=w89, "Ctl Refs in"=w87) -> ("error out"=w82:errorcluster)  [unwired: 6 in, 1 out]
  }
  n196 = disable-structure shown="Default" {
    disable-tunnel: w43 -> [_ _]
    frame condition #0 {
      n197 = Quit LabVIEW() -> ()  [unwired: 1 in]
    }
    frame condition #1 (active) {
    }
  }
